vi "Test Create Formatter.vi"(8 "error in":errorcluster) -> (0 "error out":errorcluster)   [LabVIEW 2016, in "UT_JSONLFormatter.lvlib"]
doc: "Test creation of the JSONL formatter and adding it to Handler."
uses:
  UT_JSONLFormatter.lvlib
  Source/HSE-Logger/LogLevel.ctl
  Source/HSE-Logger/Formatter/JSONLFormatter/JSONLFormatter.lvclass
  C:/Users/admin/_Git/hse-logger/Source/HSE-Logger/Formatter/Formatter.lvclass
  Source/HSE-Logger/Handler/FileHandler/FileHandler.lvclass/FileHandler.ctl
  Source/HSE-Logger/Handler/FileHandler/FileHandler.lvclass
  <vilib>/addons/_JKI Toolkits/Caraya/classes/Test/Test.lvclass
  Source/HSE-Logger/hse-logger.lvlib
  <vilib>/addons/_JKI Toolkits/Caraya/classes/Assert/Assert.lvclass
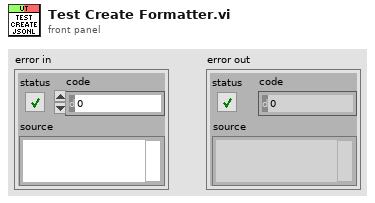
[diagram p1: front panel]
types:
  T1 = typedef "hse-logger.lvlib/LogLevel.ctl" = enum16{"DEBUG", "INFO", "WARNING", "ERROR", "CRITICAL"}
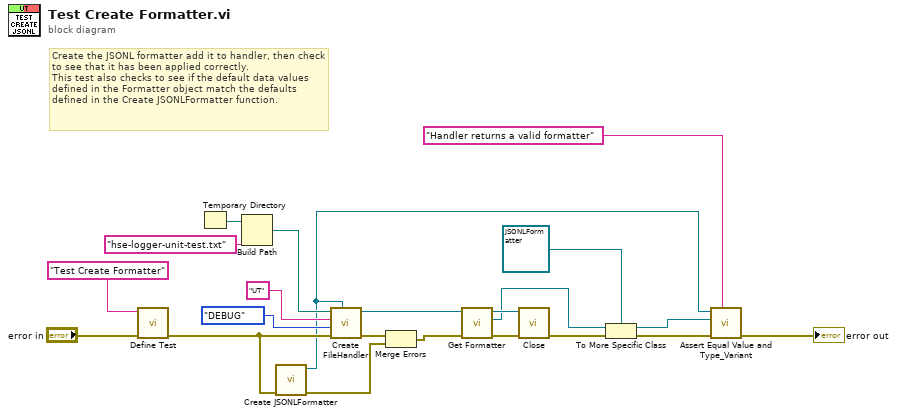
[diagram p0: block diagram]
diagram:
  # "Create the JSONL formatter add it to handler, then check to see that it has been applied correctly.\nThis test also checks to see if the default data values defined in the Formatter object match the defaults defined in the Create JSONLFormatter function."
  n1 = call <vilib>:"Define Test.vi"("error in (no error)"="error in", "Label (VI Title)"="Test Create Formatter") -> ("error out"=w11:errorcluster)  [unwired: 8 in, 1 out]
  n2 = Temporary Directory() -> (w13:path)
  n3 = Build Path(base path=w13, name or relative path="hse-logger-unit-test.txt") -> (appended path=w7:path)
  n4 = call "Create JSONLFormatter.vi"("error in"=w11) -> ("error out"=w20:errorcluster, "JSONLFormatter out"=w6:refnum<class "JSONLFormatter.lvclass">)  [unwired: 9 in]
  n5 = call "Create FileHandler.vi"("Formatter.lvclass"=w6, "error in"=w11, "Level"=LogLevel."DEBUG", "Name"="UT", "Filepath"=w7) -> ("error out"=w10:errorcluster, "FileHandler out"=w3:refnum<class "FileHandler.lvclass">)  [unwired: 5 in]
  n6 = Merge Errors(w10, w20) -> (w5:errorcluster)
  n7 = call "Get Formatter.vi"("error in"=w5, "FileHandler"=w3) -> ("error out"=w4:errorcluster, "Formatter"=w1:refnum<class "Formatter.lvclass">, "FileHandler out"=w2:refnum<class "FileHandler.lvclass">)  [unwired: 7 in]
  n8 = call-dynamic "Close.vi"("error in"=w4, "FileHandler in"=w2) -> ("error out"=w19:errorcluster)  [unwired: 8 in, 1 out]
  n9 = To More Specific Class(target class=refnum<class "JSONLFormatter.lvclass"> refnum ("hse-logger.lvlib:JSONLFormatter.lvclass"), reference=w1, error in=w19) -> (specific class reference=w15:refnum<class "JSONLFormatter.lvclass">, error out=w18:errorcluster)
  n10 = call <vilib>:"Assert Equal Value and Type_Variant.vi"("Label"="Handler returns a valid formatter", "error in (no error)"=w18, "Y"=w15, "X"=w6) -> ("error out"=→"error out":errorcluster)  [unwired: 6 in, 1 out]
